vi "Load DataBuffer.vi"(0 "Read#":u16(slide)=1 min=1 max=45 step=1 scale=1.0..45.0, 7 "File Info Buffer Init":T1[](array[typedef]) {"CCD Parameters"."dt or s" format="%#.6f"; "CCD Parameters"."Repetition" min=1; "CCD Parameters"."Offset" format="%#.2f"; "CCD Parameters"."Exposure Time (s)" min=0.02 max=6000.0 format="%#.2f"; "Center nm" format="%.2f"; "Temperature (K)" format="%.2f"; "Field (T)" format="%.2f"}, 11 "Y Array Buffer Init":dbl[][](array[numeric])=array1025x10[10250 elements] format="%.2f") -> (3 "File Info Out":T1={"FilePath"=path "/DATA/Labview Items", "Field (T)"=55.0, "Temperature (K)"=77.0, "X-Axis"=enum."nm", "Center nm"=55.0, "Current Grating Density"=enum."600", "CCD Parameters"={"Exposure Time (s)"=0.2, "Offset"=0.0, "BkgrdCrct"=FALSE, "Shutter"=FALSE, "Mode"=enum."Regular", "Repetition"=4, "dt or s"=0.0}, "Operation Mode"=enum."NML Data Acquisition", "Exp Index"=0, "Index_repetition"=0, "Index"=0, "Current Detector"=enum."CCD-1024x256"} {"CCD Parameters"."dt or s" format="%#.6f"; "CCD Parameters"."Repetition" min=1; "CCD Parameters"."Offset" format="%#.2f"; "CCD Parameters"."Exposure Time (s)" min=0.02 max=6000.0 format="%#.2f"; "Center nm" format="%.2f"; "Temperature (K)" format="%.2f"; "Field (T)" format="%.2f"}, 4 "X-Data out":dbl[](array[numeric]) format="%.2f", 6 "Y-Data out":dbl[](array[numeric]) format="%.2f", 8 "X-Axis":i32(ring)=1 items=["Point #", "nm", "eV", "meV", "cm-1"], 10 "File Info Buffer Out":T1[](array[typedef]) {"CCD Parameters"."dt or s" format="%#.6f"; "CCD Parameters"."Repetition" min=1; "CCD Parameters"."Offset" format="%#.2f"; "CCD Parameters"."Exposure Time (s)" min=0.02 max=6000.0 format="%#.2f"; "Center nm" format="%.2f"; "Temperature (K)" format="%.2f"; "Field (T)" format="%.2f"}, 14 "Continue?":bool, 15 "Y Array Buffer Out":dbl[][](array[numeric]) format="%.2f")   [LabVIEW 2020]
doc: "Write (FIFO) or retrieve (LIFO) data from the buffer.\n\nWhen write to the buffer, set the desired \"Buffer Size\" and run the VI several iterations. Notice that initially, the buffer grows to reach \"Buffer Size\" and then the input data flows from the last buffer element through to the zero element on each iteration (First In, First Out).\n\nWhen read from the buffer, set the Read# to the nth previous input data, i.e. counting reversely, with the most recent input counted as the 1st readout. If the input is out of current buffer size, an error is returned. (Last In, First Out)"
uses:
  Globals and TypeDefs/Type Definitions.llb/FileInfoParameter.ctt
  Globals and TypeDefs/Type Definitions.llb/Wavelength Unit.ctt
  Globals and TypeDefs/Type Definitions.llb/McPherson Grating Density.ctl
  Globals and TypeDefs/Type Definitions.llb/CCDParameter.ctt
  Globals and TypeDefs/Type Definitions.llb/OperationMode.ctt
  Globals and TypeDefs/Type Definitions.llb/ListOfDetectors.ctt
  File and save/X-Axis_Generator_morph.vi
panel:
  in  "continue2":bool=TRUE
  in  "Speed":u16(slide)=100 min=50 max=5000 step=50 scale=10.0..5000.0
  in  "Movie":bool
  out "File Contents":string
  in  "WL unit":i32(ring)=1 items=["Wavelength", "nm", "eV", "meV", "cm-1"]
  in  "Continue?":bool
  in  "Cancel":bool
  out "File Path":path
  out "?":T7(graph)
  # "Latest"
  # "Erliest"
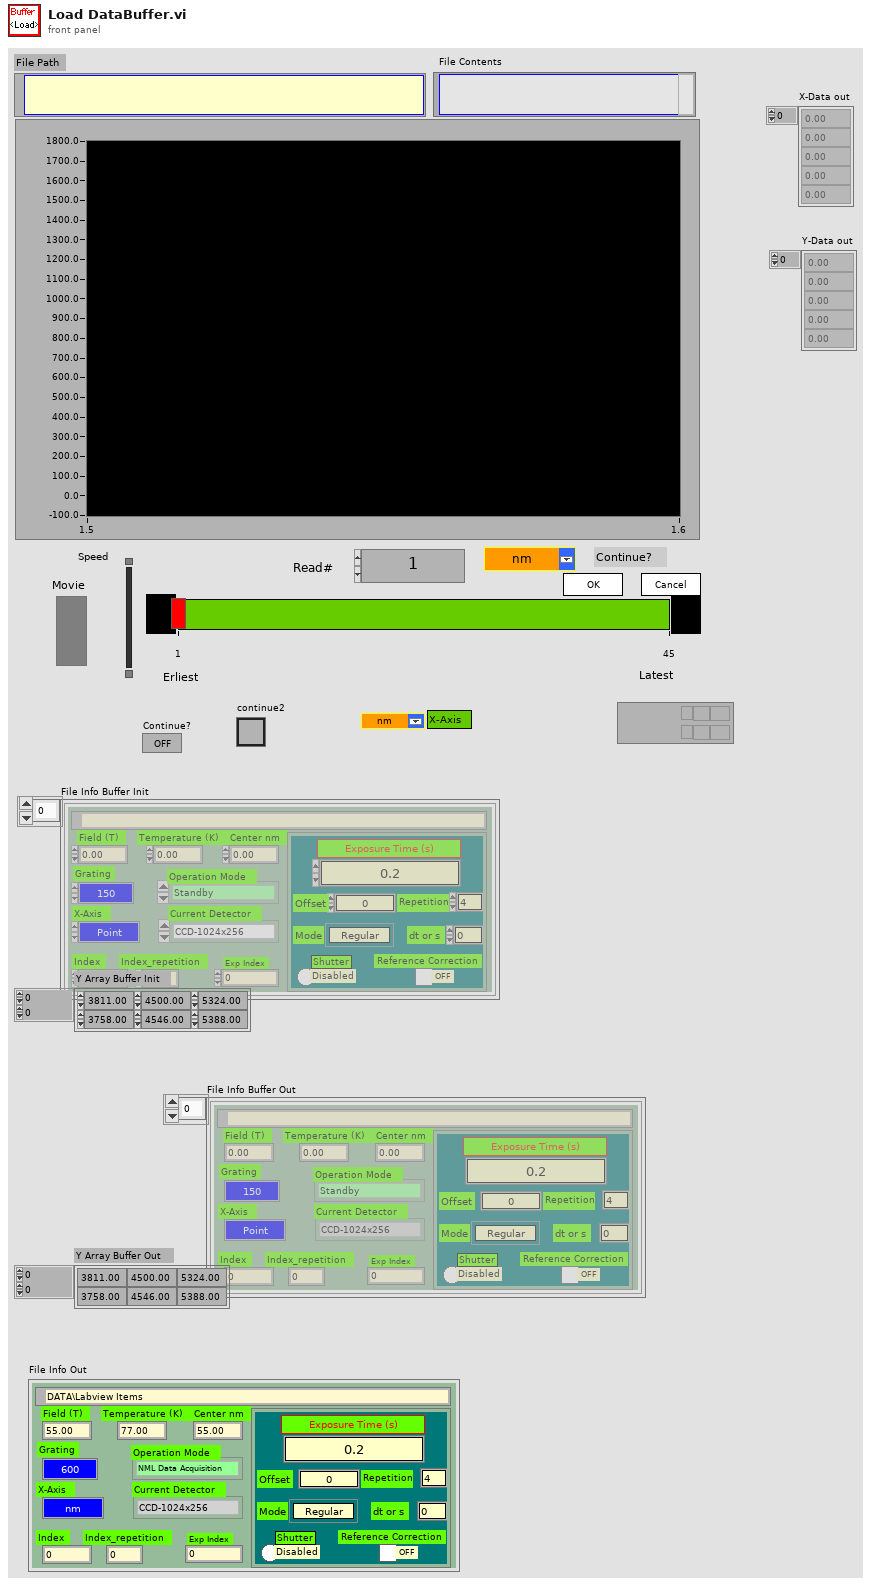
[diagram p1: front panel]
types:
  T1 = typedef "FileInfoParameter.ctt" = cluster{"FilePath":path, "Field (T)":dbl, "Temperature (K)":dbl, "X-Axis":T2, "Center nm":dbl, "Current Grating Density":T3, "CCD Parameters":T4, "Operation Mode":T5, "Exp Index":u32, "Index_repetition":u16, "Index":u16, "Current Detector":T6}
  T2 = typedef "Wavelength Unit.ctt" = enum8{"Point", "nm", "eV", "meV", "cm_1"}
  T3 = typedef "McPherson Grating Density.ctl" = enum8{"150", "300", "600", "1200", "1800"}
  T4 = typedef "CCDParameter.ctt" = cluster{"Exposure Time (s)":dbl, "Offset":dbl, "BkgrdCrct":bool, "Shutter":bool, "Mode":enum8{"Regular", "OverExp Cor", "SpikeRemove", "ForCalibration"}, "Repetition":u16, "dt or s":dbl}
  T5 = typedef "OperationMode.ctt" = enum16{"Standby", "CCD Single Shot", "CCD Sequence Shots", "CCD Custom Shots", "CCD Reference Shot", "Step Scanning ", "Time Scanning", "NML Data Acquisition"}
  T6 = typedef "ListOfDetectors.ctt" = enum8{"CCD-1024x256", "InGaAs PDA-1024x1", "CCD-1340x400", "Ge Single Channel", "Si Single Channel", "PMT Single Channel"}
  T7 = cluster{"Ramp Pattern":dbl[], "Sinc Pattern":dbl[]}
  T8 = enum16{"Pass", "Write", "Read", "ReadPlotBlock", "Initialize", "InitFromBufferInput", "Resize Buffer"}
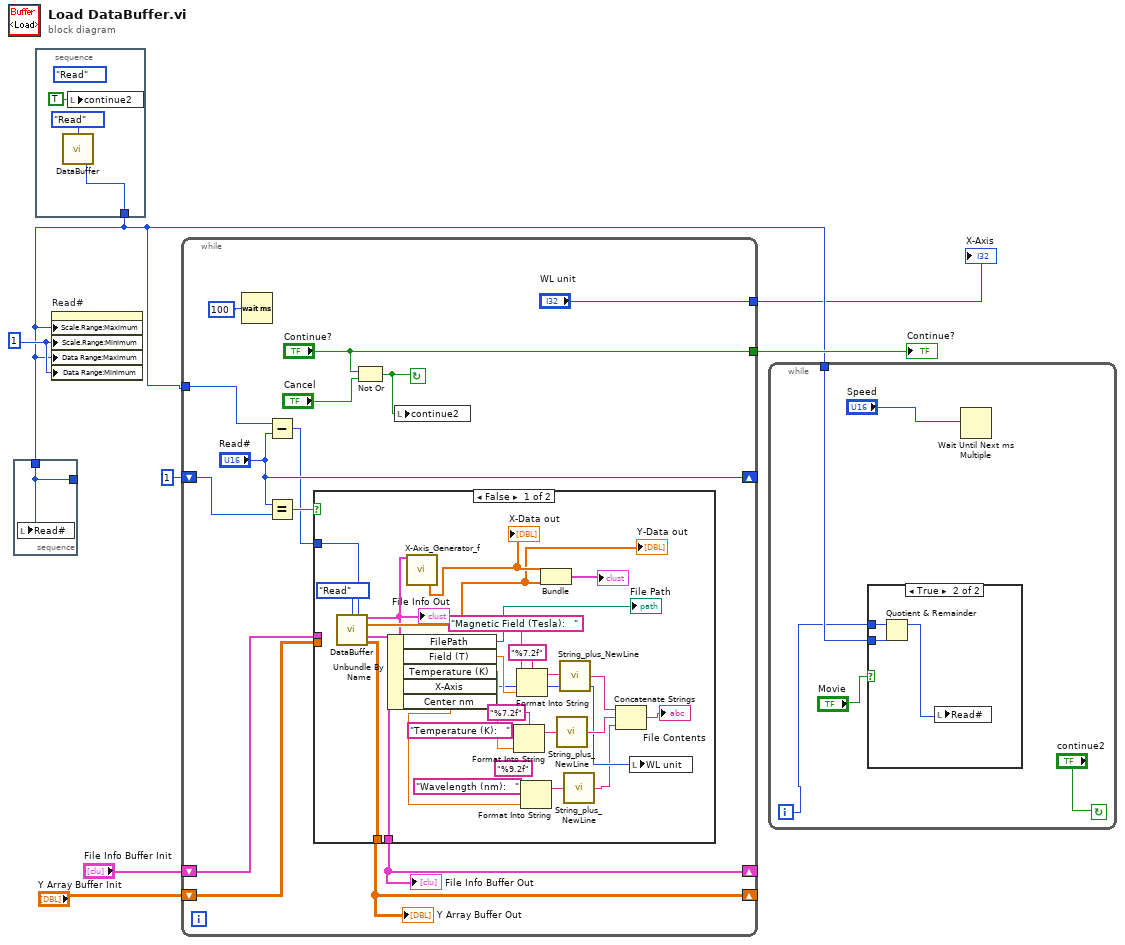
[diagram p0: block diagram]
diagram:
  w5 = u32 1 ("milliseconds to wait")
  n1 = stacked-sequence {
    tunnel: [w9] -> w4
    frame #0 {
      (unwired) enum16{"Pass", "Write", "Read", "Initialize"}."Read" ("Action")
      n2 = call "DataBuffer.vi"("Action"=T8."Read") -> ("Current Buffer Size"=w9:i32)  [unwired: 10 in, 4 out]
      n3 = local write "continue2"(TRUE ("Boolean")) -> ()
    }
  }
  n4 = stacked-sequence {
    tunnel: w4 -> [w11]
    tunnel: [w11] -> _
    frame #0 {
      n5 = local write "Read#"(w11) -> ()
    }
  }
  n6 = property on="Read#" class="Slide (strict)"("Scale.Range:Maximum"=w4, "Scale.Range:Minimum"=w5, "Data Range:Maximum"=w4, "Data Range:Minimum"=w5) -> ()  [unwired: 2 in, 2 out]
  n7 = while {
    tunnel: w4 -> [w20]
    shift-left: u8 1 ("Read#") -> [w22]
    shift-right: ["Read#"] -> _
    tunnel: ["Continue?"] -> w7
    tunnel: ["WL unit"] -> w3
    shift-right: [w13] -> _
    shift-left: "File Info Buffer Init" -> [w15]
    shift-right: [w12] -> _
    shift-left: "Y Array Buffer Init" -> [w14]
    stop <- w17 continue-if-true
    n8 = Wait (ms)(milliseconds to wait=u32 100) -> ()  [unwired: 1 out]
    n9 = Subtract(x=w20, y="Read#") -> (x-y=w18:i32)
    n10 = Equal?(x="Read#", y=w22) -> (x = y?=w21:bool)
    n11 = case shown="False" w21 {
      tunnel: w18 -> [w40 _]
      tunnel: w15 -> [_ w52]
      tunnel: w14 -> [_ w51]
      tunnel: [w33 w52] -> w13
      tunnel: [w32 w51] -> w12
      frame False {
        (unwired) "%9.2f"
        n12 = call "DataBuffer.vi"("Action"=T8."Read", "Read#"=w40) -> ("File Info Out"=w37:T1, "Y Array out"=w38:dbl[], "File Info Buffer Out"=w33:T1[], "Y Array Buffer Out"=w32:dbl[][])  [unwired: 9 in, 1 out]
        "Y-Data out" <- w38
        "File Info Out" <- w37
        n13 = Unbundle By Name(w37) -> ("FilePath"=→"File Path":path, "Field (T)"=w35:dbl, "Temperature (K)"=w34:dbl, "X-Axis"=w31:T2, "Center nm"=w27:dbl)
        n14 = call-poly "X-Axis_Generator_f.vi"("File Info In"=w37) -> ("X-axis"=w39:dbl[])  [unwired: 11 in, 7 out]
        "X-Data out" <- w39
        n15 = Format Into String(format string="%7.2f", initial string="Temperature (K):   ", w34) -> (resulting string=w46:string)  [unwired: 1 in, 1 out]
        n16 = Format Into String(format string="%7.2f", initial string="Magnetic Field (Tesla):   ", w35) -> (resulting string=w48:string)  [unwired: 1 in, 1 out]
        n17 = Format Into String(initial string="Wavelength (nm):   ", w27) -> (resulting string=w29:string)  [unwired: 2 in, 1 out]
        n18 = Bundle("X-axis"=w39, "Y Array out"=w38) -> (→"?":cluster{"X-axis":dbl[], "Y Array out":dbl[]})  [unwired: 1 in]
        n19 = call "String_plus_NewLine.vi"("Input String"=w46) -> ("Input String +[\\n]"=w42:string)
        n20 = call "String_plus_NewLine.vi"("Input String"=w48) -> ("Input String +[\\n]"=w43:string)
        n21 = call "String_plus_NewLine.vi"("Input String"=w29) -> ("Input String +[\\n]"=w26:string)
        n22 = Concatenate Strings(w43, w42, w26) -> (→"File Contents":string)
        n23 = local write "WL unit"(w31) -> ()
      }
      frame True {
      }
    }
    "Y Array Buffer Out" <- w12
    "File Info Buffer Out" <- w13
    n24 = Not Or(1:"Cancel", 2:"Continue?") -> (0:w17:bool)
    n25 = local write "continue2"(w17) -> ()
  }
  "Continue?" <- w7
  "X-Axis" <- w3
  n26 = while {
    tunnel: w4 -> [w57]
    i -> [w54]
    stop <- "continue2" continue-if-true
    n27 = case shown="True" "Movie" {
      tunnel: w57 -> [_ w60]
      tunnel: w54 -> [_ w58]
      frame False {
      }
      frame True {
        n28 = Quotient & Remainder(x=w58, y=w60) -> (x-y*floor(x/y)=w59:i32)  [unwired: 1 out]
        n29 = local write "Read#"(w59) -> ()
      }
    }
    n30 = Wait Until Next ms Multiple(millisecond multiple="Speed") -> ()  [unwired: 1 out]
  }
